vi "clusterexperiment.vi"() -> ()   [LabVIEW 2014]
panel:
  out "Small Cluster":cluster{"Boolean":bool, "Slide value":dbl}
  out "Modified Cluster":T1 {"Slide" scale=0.0..10.0}
  in  "Cluster":T1 {"Slide" scale=0.0..10.0}
  out "Boolean 2":bool
  out "Numeric":dbl
  in  "stop":bool
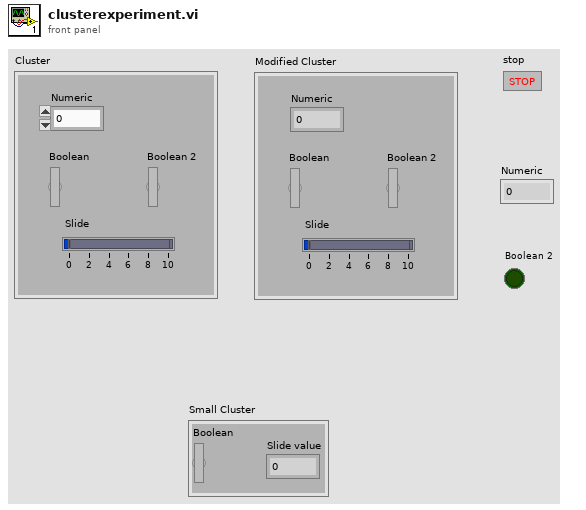
[diagram p1: front panel]
types:
  T1 = cluster{"Numeric":dbl, "Boolean":bool, "Boolean 2":bool, "Slide":dbl}
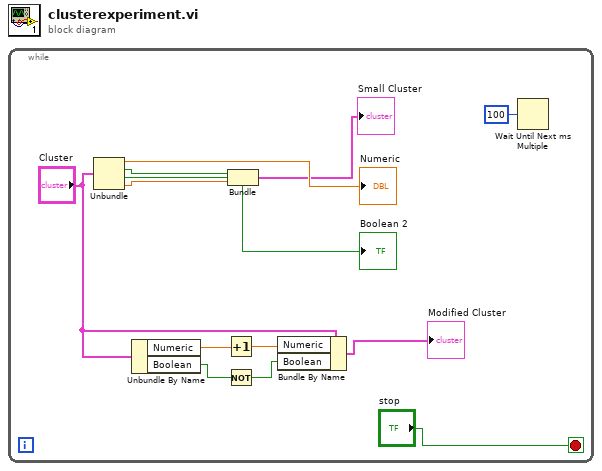
[diagram p0: block diagram]
diagram:
  n1 = while {
    stop <- "stop" stop-if-true
    n2 = Unbundle("Cluster") -> ("Numeric"=→"Numeric":dbl, "Boolean"=w12:bool, "Boolean 2"=→"Boolean 2":bool, "Slide"=w13:dbl)
    n3 = Unbundle By Name("Cluster") -> ("Numeric"=w8:dbl, "Boolean"=w7:bool)
    n4 = Increment(x=w8) -> (x+1=w5:dbl)
    n5 = Not(x=w7) -> (.not. x?=w4:bool)
    n6 = Bundle("Boolean"=w12, "Slide"=w13) -> (→"Small Cluster":cluster{"Boolean":bool, "Slide":dbl})  [unwired: 1 in]
    n7 = Bundle By Name(cluster="Cluster", "Numeric"=w5, "Boolean"=w4) -> (→"Modified Cluster":T1)
    n8 = Wait Until Next ms Multiple(millisecond multiple=u32 100) -> ()  [unwired: 1 out]
  }
